vi "Alarm Model to UI Alarm.vi"(11 "Alarm Model":T2={"Color Box"=16777226, "Name"="TT1:Lo", "Ack"=FALSE, "Alarm"={"alarm URL"="\\\\.\\Pfizer FAST\\TT1.Alarms.TT1:Lo", "set time"=timestamp(3634824639.8324924 s since 1904-01-01), "set user"="(Nobody)", "ack time"=timestamp(-9223372036854775808 s since 1904-01-01), "ack user"="", "clear time"=timestamp(-9223372036854775808 s since 1904-01-01), "clear user"="", "setpoint"=30.0, "value"=22.498404260798484, "priority"=1, "alarm area"="", "alarm description"="", "ack comment"="", "event?"=FALSE, "Refnum"=216172782113783883}} {"Alarm"."value" format="%.2f"; "Alarm"."setpoint" format="%.2f"; "Alarm"."clear time" format="%<%X\n%x>T"; "Alarm"."ack time" format="%<%X\n%x>T"; "Alarm"."set time" format="%<%X\n%x>T"}) -> (3 "UI Alarm":T1)   [LabVIEW 2018, in "Dynamic Shared Variables.lvlib"]
doc: "Converts internal \"model\" representation of the alarm to the strict typdef used on the UI"
uses:
  Dynamic Shared Variables.lvlib
  Alarm Cluster.ctl
  Alarm Cluster (UI).ctl
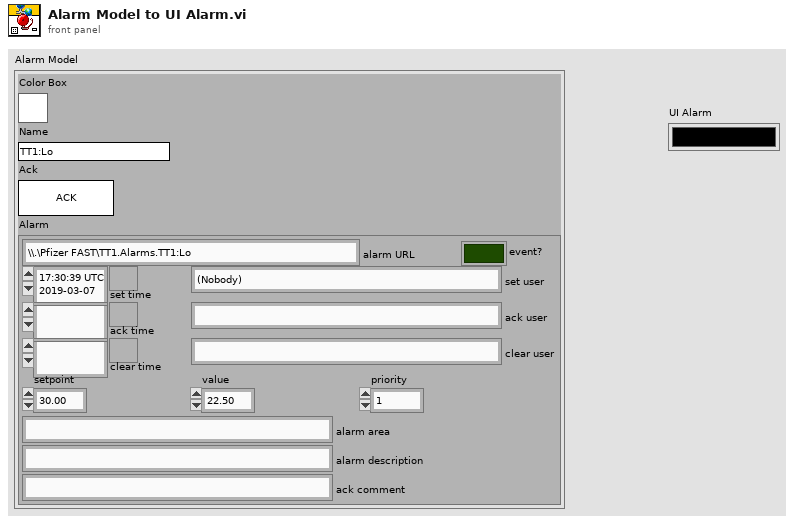
[diagram p1: front panel]
types:
  T1 = typedef "Dynamic Shared Variables.lvlib/Alarm Cluster (UI).ctl" = cluster{"Color Box":u32, "Name":string, "Ack":bool}
  T2 = typedef "Dynamic Shared Variables.lvlib/Alarm Cluster.ctl" = cluster{"Color Box":u32, "Name":string, "Ack":bool, "Alarm":cluster{"alarm URL":string, "set time":timestamp, "set user":string, "ack time":timestamp, "ack user":string, "clear time":timestamp, "clear user":string, "setpoint":dbl, "value":dbl, "priority":u32, "alarm area":string, "alarm description":string, "ack comment":string, "event?":bool, "Refnum":u64}}
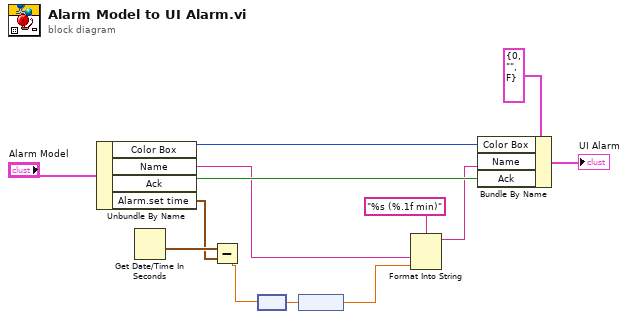
[diagram p0: block diagram]
diagram:
  n1 = Unbundle By Name("Alarm Model") -> ("Color Box"=w10:u32, "Name"=w5:string, "Ack"=w9:bool, "Alarm.set time"=w6:timestamp)
  n2 = Get Date/Time In Seconds() -> (seconds since 1Jan1904=w7:timestamp)
  n3 = Subtract(x=w7, y=w6) -> (x-y=w2:dbl)
  n4 = node(w2) -> (w3:dbl[unit])
  n5 = node(w3) -> (w1:dbl)
  n6 = Format Into String(format string="%s (%.1f min)", w5, w1) -> (resulting string=w4:string)  [unwired: 2 in, 1 out]
  n7 = Bundle By Name(cluster=T1 {"Color Box"=0, "Name"="", "Ack"=FALSE} ("UI Alarm"), "Color Box"=w10, "Name"=w4, "Ack"=w9) -> (→"UI Alarm":T1)
